vi "Close.vi"(8 "error in (no error)":errorcluster, 11 "IMAQdx Camera in":refnum<class "IMAQdx Camera.lvclass">) -> (0 "error out":errorcluster, 3 "IMAQdx Camera out":refnum<class "IMAQdx Camera.lvclass">)   [LabVIEW 2011, in "IMAQdx Camera.lvclass"]
uses:
  IMAQdx Camera.lvclass
  <vilib>/userdefined/High Color/IMAQdx.ctl
  IMAQdx Camera.lvclass/IMAQdx Camera.ctl
  <vilib>/vision/driver/NI_Vision_Acquisition_Software.lvlib
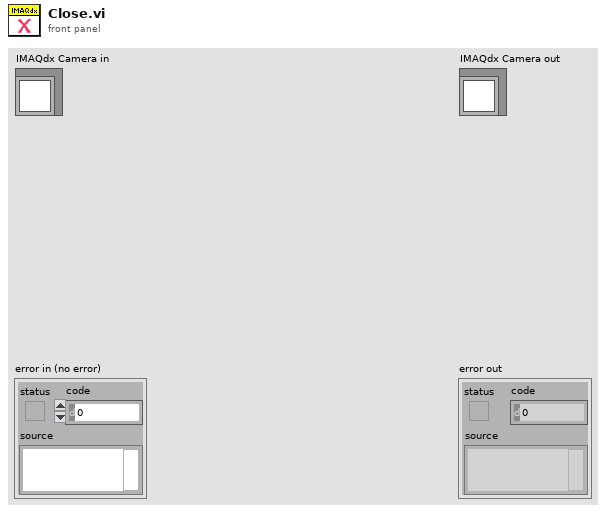
[diagram p1: front panel]
types:
  T1 = typedef "IMAQdx.ctl" = refnum<k21>
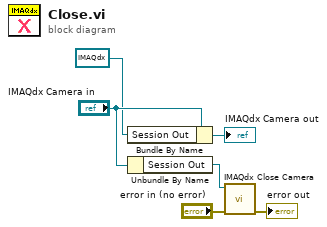
[diagram p0: block diagram]
diagram:
  n1 = Bundle By Name(cluster="IMAQdx Camera in", "Session Out"=T1 refnum) -> (→"IMAQdx Camera out":refnum<class "IMAQdx Camera.lvclass">)
  n2 = Unbundle By Name("IMAQdx Camera in") -> ("Session Out"=w5:T1)
  n3 = call <vilib>:"IMAQdx Close Camera.vi"("error in"="error in (no error)", "Session In"=w5) -> ("error out"=→"error out":errorcluster)  [unwired: 9 in]
